vi "AC2250 Measurement Mode.vi"(7 "Term Char":enum16{"Cr/Lf"}(ring), 8 "ErrIn":errorcluster, 10 "Measurement Mode":T1(ring), 11 "VISA Resource Name In":refnum<visa-resource-name>) -> (0 "ErrOut":errorcluster, 2 "Return Count":i32, 3 "VISA Resource Name Out":refnum<visa-resource-name>)   [LabVIEW 2013]
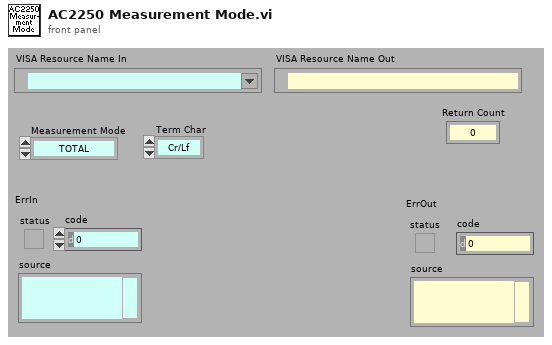
[diagram p1: front panel]
types:
  T1 = enum16{"TOTAL", "FUNDAMENTAL", "IN PHASE", "QUADRATURE", "PHASE ANGLE", "THD"}
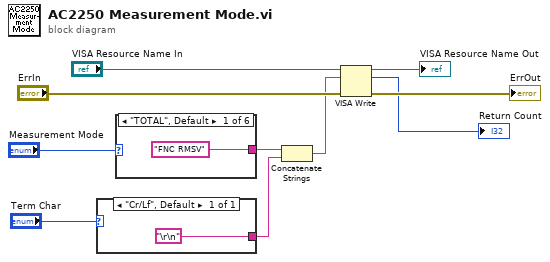
[diagram p0: block diagram]
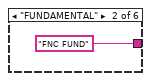
[diagram p2: hidden frame]
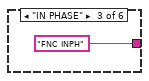
[diagram p3: hidden frame]
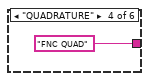
[diagram p4: hidden frame]
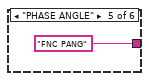
[diagram p5: hidden frame]
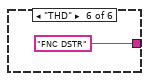
[diagram p6: hidden frame]
diagram:
  n1 = case shown="\"Cr/Lf\", Default" "Term Char" {
    tunnel: ["\r\n"] -> w3
    frame "Cr/Lf", Default {
    }
  }
  n2 = case shown="\"TOTAL\", Default" "Measurement Mode" {
    tunnel: ["FNC RMSV" "FNC FUND" "FNC INPH" "FNC QUAD" "FNC PANG" "FNC DSTR"] -> w5
    frame "TOTAL", Default {
    }
    frame "FUNDAMENTAL" {
    }
    frame "IN PHASE" {
    }
    frame "QUADRATURE" {
    }
    frame "PHASE ANGLE" {
    }
    frame "THD" {
    }
  }
  n3 = Concatenate Strings(w5, w3) -> (w2:string)
  n4 = VISA Write(VISA resource name="VISA Resource Name In", write buffer=w2, error in (no error)="ErrIn") -> (VISA resource name out=→"VISA Resource Name Out":refnum<visa-resource-name>, return count=→"Return Count":u32, error out=→"ErrOut":errorcluster)
